vi "Write SampleRate.vi"(8 "error in (no error)":errorcluster, 10 "SampleRate":dbl, 11 "ArbitraryFunction in":refnum<class "ArbitraryFunction.lvclass">) -> (0 "error out":errorcluster, 3 "ArbitraryFunction out":refnum<class "ArbitraryFunction.lvclass">)   [LabVIEW 2018, in "Functions.lvlib" / "ArbitraryFunction.lvclass"]
uses:
  ArbitraryFunction.lvclass
  ArbitraryFunction.lvclass/ArbitraryFunction.ctl
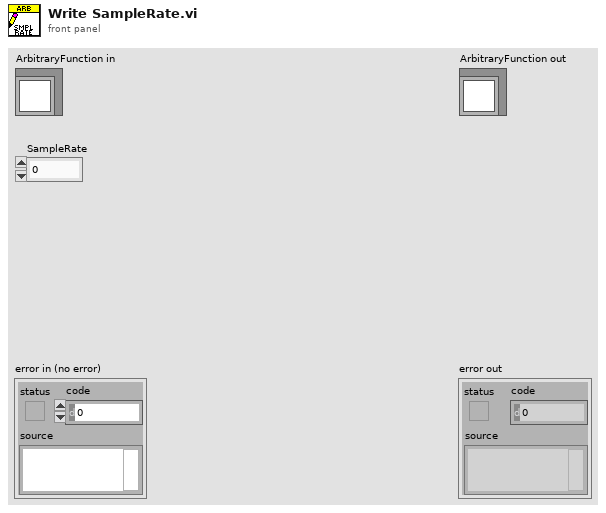
[diagram p1: front panel]
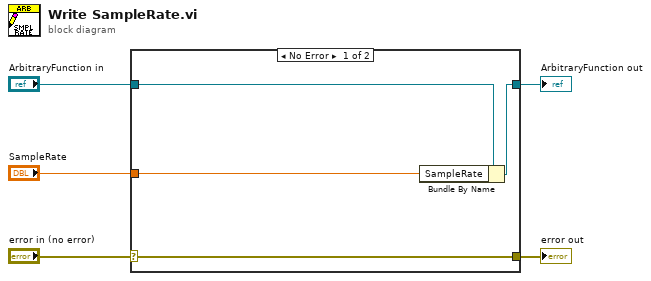
[diagram p0: block diagram]
diagram:
  n1 = case shown="No Error" "error in (no error)" {
    selector: "error in (no error)" -> [w9 w10]
    tunnel: [w9 w10] -> w4
    tunnel: [w7 w11] -> w2
    tunnel: "ArbitraryFunction in" -> [w8 w11]
    tunnel: "SampleRate" -> [w6 _]
    frame No Error {
      n2 = Bundle By Name(cluster=w8, "SampleRate"=w6) -> (w7:refnum<class "ArbitraryFunction.lvclass">)
    }
    frame Error {
    }
  }
  "error out" <- w4
  "ArbitraryFunction out" <- w2
